vi "NI_Init.vi"(5 "error in (no error)":errorcluster, 7 "Analog input sampling time (s)":dbl, 8 "Olfactometer parameters":T1={"Back valve ON delays"=[0.0, 0.0, 0.0, 0.0, 0.0, 0.0, 0.0, 0.0, 0.0, 0.0, 0.0, 0.0, 0.0, 0.0, 0.0, 0.0], "Back valve OFF delays"=[0.0, 0.0, 0.0, 0.0, 0.0, 0.0, 0.0, 0.0, 0.0, 0.0, 0.0, 0.0, 0.0, 0.0, 0.0, 0.0], "Step duration (ms)"=2.0, "TTL binary step duration (ms)"=1.0, "Sampling rate (Hz)"=20000.0, "Initial delay (ms)"=0.0, "Pulse duration (ms)"=250.0} {"Initial delay (ms)" format="%#_13g"}) -> (0 "error out":errorcluster, 3 "NI cluster out":T3={"AI task out"="", "DO task out"="", "AI samples"=0, "Olfactometer parameters"={"Back valve ON delays"=[0.0, 0.0, 0.0, 0.0, 0.0, 0.0, 0.0, 0.0, 0.0, 0.0, 0.0, 0.0, 0.0, 0.0, 0.0, 0.0], "Back valve OFF delays"=[0.0, 0.0, 0.0, 0.0, 0.0, 0.0, 0.0, 0.0, 0.0, 0.0, 0.0, 0.0, 0.0, 0.0, 0.0, 0.0], "Step duration (ms)"=2.0, "TTL binary step duration (ms)"=1.0, "Sampling rate (Hz)"=20000.0, "Initial delay (ms)"=500.0, "Pulse duration (ms)"=500.0}})   [LabVIEW 2016]
uses:
  NI_cluster.ctl
  <vilib>/DAQmx/create/channels.llb/DAQmx Create Channel (AI-Voltage-Basic).vi
  <vilib>/DAQmx/configure/timing.llb/DAQmx Timing (Sample Clock).vi
  <vilib>/DAQmx/create/channels.llb/DAQmx Create Channel (DO-Digital Output).vi
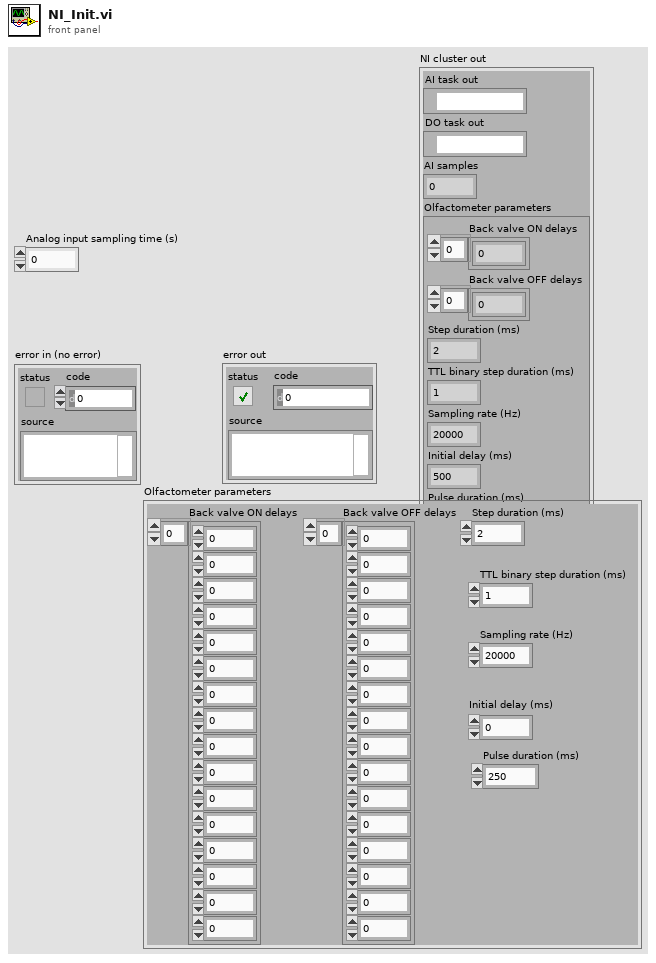
[diagram p1: front panel]
types:
  T1 = cluster{"Back valve ON delays":dbl[], "Back valve OFF delays":dbl[], "Step duration (ms)":dbl, "TTL binary step duration (ms)":dbl, "Sampling rate (Hz)":dbl, "Initial delay (ms)":dbl, "Pulse duration (ms)":dbl}
  T2 = typedef "NI_cluster.ctl" = refnum<k21>
  T3 = cluster{"AI task out":refnum<k21>, "DO task out":T2, "AI samples":i32, "Olfactometer parameters":cluster{"Back valve ON delays":dbl[], "Back valve OFF delays":dbl[], "Step duration (ms)":dbl, "TTL binary step duration (ms)":dbl, "Sampling rate (Hz)":dbl, "Initial delay (ms)":dbl, "Pulse duration (ms)":dbl}}
  T4 = cluster{"Initial phase":i32, "Back-valve pre-phase ":i32, "Main phase":i32, "Back-valve post-phase":i32, "Reset":i32, "Step":i32, "Total":i32, "ON delays":i32[], "OFF delays":i32[]}
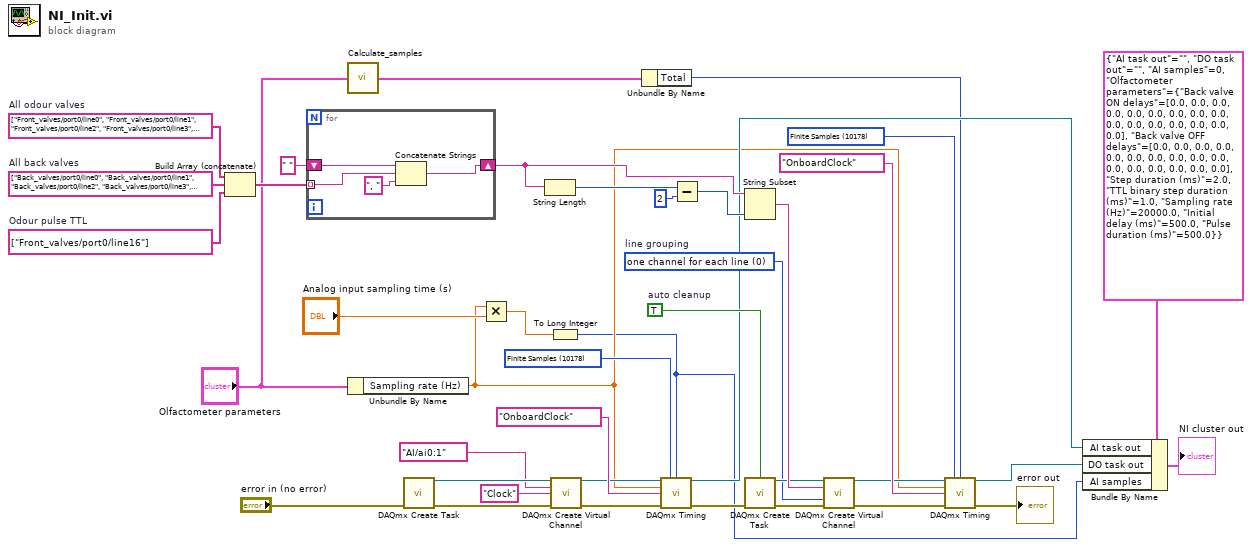
[diagram p0: block diagram]
diagram:
  w9 = 10178 items=["Finite Samples"=10178, "Continuous Samples"=10123, "Hardware Timed Single Point"=12522] ("sample mode")
  w40 = 10178 items=["Finite Samples"=10178, "Continuous Samples"=10123, "Hardware Timed Single Point"=12522] ("sample mode")
  w38 = tag[] ["Back_valves/port0/line0", "Back_valves/port0/line1", "Back_valves/port0/line2", "Back_valves/port0/line3", "Back_valves/port0/line4", "Back_valves/port0/line5", "Back_valves/port0/line6", "Back_valves/port0/line7", "Back_valves/port0/line16", "Back_valves/port0/line17", "Back_valves/port0/line18", "Back_valves/port0/line19", "Back_valves/port0/line20", "Back_valves/port0/line21", "Back_valves/port0/line22", "Back_valves/port0/line23"]  # All back valves
  w37 = tag[] ["Front_valves/port0/line0", "Front_valves/port0/line1", "Front_valves/port0/line2", "Front_valves/port0/line3", "Front_valves/port0/line4", "Front_valves/port0/line5", "Front_valves/port0/line6", "Front_valves/port0/line7", "Front_valves/port0/line8", "Front_valves/port0/line9", "Front_valves/port0/line10", "Front_valves/port0/line11", "Front_valves/port0/line12", "Front_valves/port0/line13", "Front_valves/port0/line14", "Front_valves/port0/line15"]  # All odour valves
  w34 = tag[] ["Front_valves/port0/line16"]  # Odour pulse TTL
  w17 = 0 items=["one channel for each line", "one channel for all lines"]  # line grouping
  w16 = TRUE  # auto cleanup
  n1 = Build Array (concatenate)(w37, w38, w34) -> (w19:tag[])
  n2 = for {
    tunnel: w19 -> [w44] mode=indexing
    shift-right: [w41] -> w21
    shift-left: " " ("concatenated string") -> [w42]
    n3 = Concatenate Strings(w42, w44, ", " ("concatenated string")) -> (w41:string)
  }
  n4 = call "Calculate_samples.vi"("Olfactormeter parameters"="Olfactometer parameters") -> ("Samples"=w11:T4)  [unwired: 4 in]
  n5 = Unbundle By Name("Olfactometer parameters") -> ("Sampling rate (Hz)"=w3:dbl)
  n6 = call <vilib>:"DAQmx Create Task.vi"("error in"="error in (no error)") -> ("task out"=w28:refnum<k21>, "error out"=w26:errorcluster)  [unwired: 13 in]
  n7 = Multiply(x=w3, y="Analog input sampling time (s)") -> (x*y=w10:dbl)
  n8 = String Length(string=w21) -> (length=w23:i32)
  n9 = To Long Integer(number=w10) -> (32bit integer=w1:i32)
  n10 = call-poly <vilib>:"DAQmx Create Virtual Channel.vi"("task in"=w28, "physical channels"=tag "AI/ai0:1", "name to assign"="Clock", "error in"=w26) -> ("task out"=w32:refnum<k21>, "error out"=w33:errorcluster)  [unwired: 10 in]
  n11 = Unbundle By Name(w11) -> ("Total"=w2:i32)
  n12 = call-poly <vilib>:"DAQmx Timing.vi"("task/channels in"=w32, "sample mode"=w40, "samples per channel"=w1, "rate"=w3, "source"=tag "OnboardClock" ("Sample Clock Source"), "error in"=w33) -> ("task out"=w13:refnum<k21>, "error out"=w31:errorcluster)  [unwired: 8 in]
  n13 = Subtract(x=w23, y=2) -> (x-y=w22:i32)
  n14 = String Subset(string=w21, length (rest)=w22) -> (substring=w25:string)  [unwired: 1 in]
  n15 = call <vilib>:"DAQmx Create Task.vi"("auto cleanup"=w16, "error in"=w31) -> ("task out"=w20:refnum<k21>, "error out"=w30:errorcluster)  [unwired: 12 in]
  n16 = call-poly <vilib>:"DAQmx Create Virtual Channel.vi"("task in"=w20, "lines"=w25, "line grouping"=w17, "error in"=w30) -> ("task out"=w7:refnum<k21>, "error out"=w5:errorcluster)  [unwired: 10 in]
  n17 = call-poly <vilib>:"DAQmx Timing.vi"("task/channels in"=w7, "sample mode"=w9, "samples per channel"=w2, "rate"=w3, "source"=tag "OnboardClock", "error in"=w5) -> ("task out"=w6:refnum<k21>, "error out"=→"error out":errorcluster)  [unwired: 8 in]
  n18 = Bundle By Name(cluster=T3 {"AI task out"="", "DO task out"="", "AI samples"=0, "Olfactometer parameters"={"Back valve ON delays"=[0.0, 0.0, 0.0, 0.0, 0.0, 0.0, 0.0, 0.0, 0.0, 0.0, 0.0, 0.0, 0.0, 0.0, 0.0, 0.0], "Back valve OFF delays"=[0.0, 0.0, 0.0, 0.0, 0.0, 0.0, 0.0, 0.0, 0.0, 0.0, 0.0, 0.0, 0.0, 0.0, 0.0, 0.0], "Step duration (ms)"=2.0, "TTL binary step duration (ms)"=1.0, "Sampling rate (Hz)"=20000.0, "Initial delay (ms)"=500.0, "Pulse duration (ms)"=500.0}}, "AI task out"=w13, "DO task out"=w6, "AI samples"=w1) -> (→"NI cluster out":T3)
